vi "Tolerance_v01.vi"(9 "Ring":u16(ring) items=["Default", "Five Best p-values"], 10 "Tolerance Threshold":dbl=0.05, 11 "parray":dbl[](array[numeric])) -> (3 "Boolean":bool)   [LabVIEW 2015]
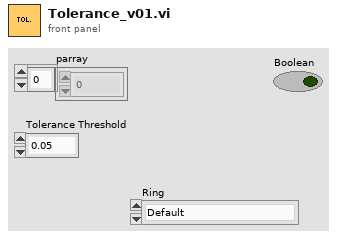
[diagram p1: front panel]
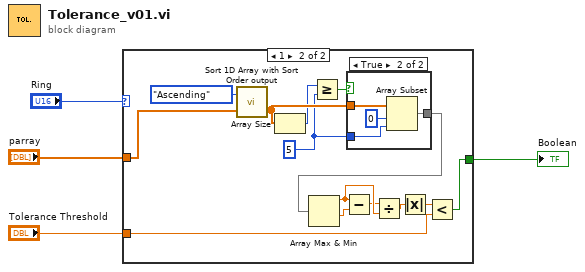
[diagram p0: block diagram]
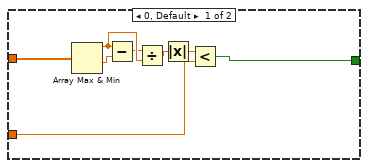
[diagram p2: hidden frame]
diagram:
  n1 = case shown="1" "Ring" {
    tunnel: [w12 w18] -> w4
    tunnel: "parray" -> [w11 w26]
    tunnel: "Tolerance Threshold" -> [w10 w19]
    frame 0, Default {
      n2 = Array Max & Min(array=w11) -> (max value=w9:dbl, min value=w5:dbl)  [unwired: 2 out]
      n3 = Subtract(x=w9, y=w5) -> (x-y=w7:dbl)
      n4 = Divide(x=w7, y=w9) -> (x/y=w8:dbl)
      n5 = Absolute Value(x=w8) -> (abs(x)=w6:dbl)
      n6 = Less?(x=w6, y=w10) -> (x < y?=w12:bool)
    }
    frame 1 {
      w14 = 5 ("length")
      n7 = call "Sort 1D Array with Sort Order output.vi"("Disordered Array"=w26, "Sort Order"=enum16{"Ascending", "Descending"}."Ascending") -> ("Ordered Array"=w16:dbl[])  [unwired: 1 out]
      n8 = Array Size(array=w16) -> (size(s)=w15:i32)
      n9 = Greater Or Equal?(x=w15, y=w14) -> (x >= y?=w13:bool)
      n10 = case shown="True" w13 {
        tunnel: w16 -> [w27 w31]
        tunnel: w14 -> [_ w29]
        tunnel: [w27 w28] -> w17
        frame False {
        }
        frame True {
          n11 = Array Subset(array=w31, index=0, length=w29) -> (w28:dbl[])
        }
      }
      n12 = Array Max & Min(array=w17) -> (max value=w24:dbl, min value=w20:dbl)  [unwired: 2 out]
      n13 = Subtract(x=w24, y=w20) -> (x-y=w22:dbl)
      n14 = Divide(x=w22, y=w24) -> (x/y=w23:dbl)
      n15 = Absolute Value(x=w23) -> (abs(x)=w21:dbl)
      n16 = Less?(x=w21, y=w19) -> (x < y?=w18:bool)
    }
  }
  "Boolean" <- w4
